vi "Refresh Max Sizes.vi"(8 "error in (no error)":errorcluster, 11 "2DArrayManager in":refnum<class "2DArrayManager.lvclass">) -> (0 "error out":errorcluster, 3 "2DArrayManager out":refnum<class "2DArrayManager.lvclass">)   [LabVIEW 2020, in "OOPanel.lvlib" / "2DArrayManager.lvclass"]
uses:
  2DArrayManager.lvclass
  2DArrayManager.lvclass/2DArrayManager.ctl
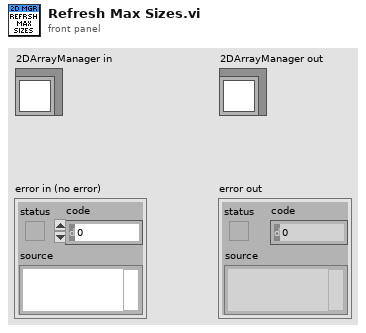
[diagram p1: front panel]
types:
  T1 = typedef "OOPanel.lvlib/Desired Size.ctl" = cluster{"Width":u32, "Height":u32}
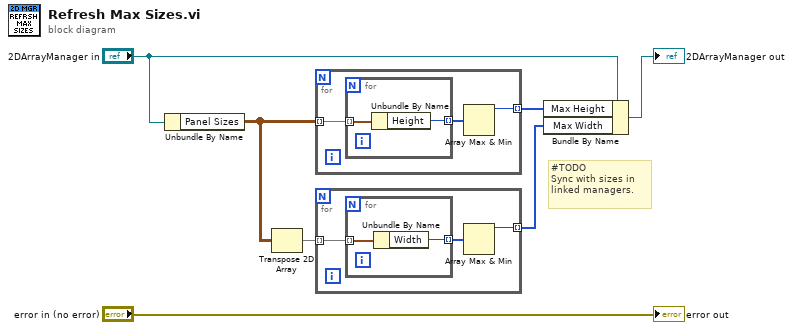
[diagram p0: block diagram]
diagram:
  # "#TODO\nSync with sizes in linked managers."
  n1 = Unbundle By Name("2DArrayManager in") -> ("Panel Sizes"=w4:T1[][])
  n2 = Transpose 2D Array(2D array=w4) -> (transposed array=w5:T1[][])
  n3 = for {
    tunnel: w4 -> [w10] mode=indexing
    tunnel: [w8] -> w2 mode=indexing
    n4 = for {
      tunnel: w10 -> [w12] mode=indexing
      tunnel: [w11] -> w9 mode=indexing
      n5 = Unbundle By Name(w12) -> ("Height"=w11:u32)
    }
    n6 = Array Max & Min(array=w9) -> (max value=w8:u32)  [unwired: 3 out]
  }
  n7 = for {
    tunnel: w5 -> [w15] mode=indexing
    tunnel: [w13] -> w1 mode=indexing
    n8 = for {
      tunnel: w15 -> [w17] mode=indexing
      tunnel: [w16] -> w14 mode=indexing
      n9 = Unbundle By Name(w17) -> ("Width"=w16:u32)
    }
    n10 = Array Max & Min(array=w14) -> (max value=w13:u32)  [unwired: 3 out]
  }
  n11 = Bundle By Name(cluster="2DArrayManager in", "Max Height"=w2, "Max Width"=w1) -> (→"2DArrayManager out":refnum<class "2DArrayManager.lvclass">)
  "error out" <- "error in (no error)"
